vi "JL_Knob Turn.vi"(0 "GEA2 Reference In":refnum<k24>, 2 "Knob Position":T1, 5 "Error In":errorcluster) -> (14 "GEA2 Reference Out":refnum<k24>, 19 "Error Out":errorcluster)   [LabVIEW 2018]
uses:
  D:/Common/DLLs/GEA3/GeaCommunication.dll
  Common/DLLs/GEA3/GeaCommunication.dll
  Type Defs/JL_Encoder_ Position.ctl
  Common/LabVIEW GEA2 Toolkit/GEA3/type defs/Source_Destination.ctl
  Common/LabVIEW GEA2 Toolkit/GEA3/type defs/ERD Write Data In.ctl
  Common/LabVIEW GEA2 Toolkit/GEA3/type defs/Data Type.ctl
  C:/Users/iallatyp/Desktop/New folder/GEA3/library/GEA2_Toolkit.lvlib
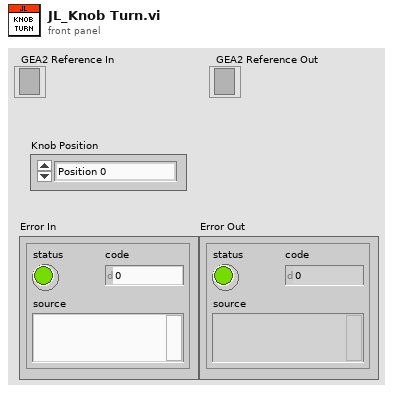
[diagram p1: front panel]
types:
  T1 = typedef "JL_Encoder_ Position.ctl" = enum16{"Position 0", "Position 1", "Position 2", "Position 3", "Position 4", "Position 5", "Position 6", "Position 7", "Position 8", "Position 9", "Position 10", "Position 11", "Position 12", "Position 13", "Position 14", "Clear / Reset"}
  T2 = typedef "GEA2_Toolkit.lvlib/ERD Write Data In.ctl" = cluster{"ERD Number":u16, "Data Type":T3, "Data":string}
  T3 = typedef "GEA2_Toolkit.lvlib/Data Type.ctl" = enum16{"string", "boolean", "uint8_t", "uint16_t", "uint32_t", "uint64_t", "int8_t", "int16_t", "int32_t", "int64_t"}
  T4 = typedef "GEA2_Toolkit.lvlib/Source_Destination.ctl" = cluster{"Source":u8, "Destination":u8}
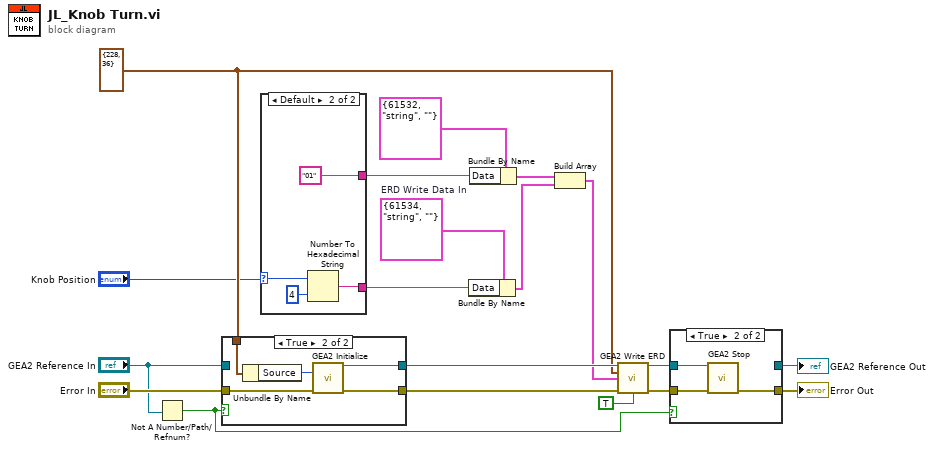
[diagram p0: block diagram]
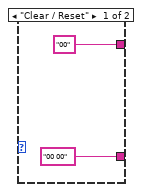
[diagram p2: hidden frame]
diagram:
  w11 = T2 {"ERD Number"=61534, "Data Type"=enum."string", "Data"=""}  # ERD Write Data In
  w13 = T4 {"Source"=228, "Destination"=36} ("GEA Inputs")
  n1 = Not A Number/Path/Refnum?(number/path/refnum="GEA2 Reference In") -> (NaN/Path/Refnum?=w3:bool)
  n2 = case shown="True" w3 {
    tunnel: "Error In" -> [w20 w26]
    tunnel: [w20 w25] -> w16
    tunnel: "GEA2 Reference In" -> [w21 _]
    tunnel: [w21 w24] -> w14
    tunnel: w13 -> [_ w22]
    frame False {
    }
    frame True {
      n3 = Unbundle By Name(w22) -> ("Source"=w23:u8)
      n4 = call "GEA2 Initialize.vi"("Source Address"=w23, "error in"=w26) -> ("GEA2 Reference Out"=w24:refnum<k24>, "error out"=w25:errorcluster)  [unwired: 11 in, 1 out]
    }
  }
  n5 = case shown="Default" "Knob Position" {
    selector: "Knob Position" -> [_ w32]
    tunnel: ["00 00" ("Message") w31] -> w10
    tunnel: ["00" ("Message") "01" ("Message")] -> w8
    frame "Clear / Reset" {
    }
    frame Default {
      n6 = Number To Hexadecimal String(1:i16 4 ("width (-)"), 2:w32) -> (0:w31:string)
    }
  }
  n7 = Bundle By Name(cluster=w11, "Data"=w10) -> (w6:T2)
  n8 = Bundle By Name(cluster=T2 {"ERD Number"=61532, "Data Type"=enum."string", "Data"=""} ("ERD Write Data In"), "Data"=w8) -> (w7:T2)
  n9 = Build Array(w7, w6) -> (w5:T2[])
  n10 = call "GEA2 Write ERD.vi"("GEA2 Reference In"=w14, "GEA Inputs"=w13, "Write ERD List"=w5, "Error In"=w16, "Verify ERD Response?"=TRUE) -> ("GEA2 Reference Out"=w12:refnum<k24>, "Error Out"=w15:errorcluster)  [unwired: 8 in, 1 out]
  n11 = case shown="True" w3 {
    tunnel: [w33 w37] -> w18
    tunnel: w12 -> [w34 w36]
    tunnel: [w34 _] -> w17
    tunnel: w15 -> [w33 w35]
    frame False {
    }
    frame True {
      n12 = call "GEA2 Stop.vi"("GEA2 Reference In"=w36, "Error In"=w35) -> ("Error Out"=w37:errorcluster)  [unwired: 13 in]
    }
  }
  "Error Out" <- w18
  "GEA2 Reference Out" <- w17
